vi "PI Id (FXP).vi"(5 "Process Value":fxp<+/-,32,4>, 7 "Setpoint":fxp<+/-,32,1>, 10 "Ki":fxp<+/-,32,4>, 11 "Kp":fxp<+/-,32,4>) -> (3 "Output":fxp<+/-,32,4> format="%.30g")   [LabVIEW 2025]
uses:
  <vilib>/rvi/FXPMathLib/FxpSub/XNode/nifxpmath_Sub.xnode
  <vilib>/rvi/FXPMathLib/sim/FxpSim.dll
  <vilib>/rvi/FXPMathLib/FxpMul/XNode/nifxpmath_Multiplier.xnode
  <vilib>/rvi/FXPMathLib/FxpAdd/XNode/nifxpmath_Add.xnode
panel:
  out "e*s":fxp<+/-,32,4> format="%.30g"
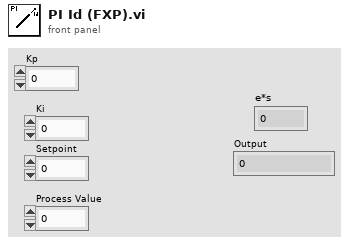
[diagram p1: front panel]
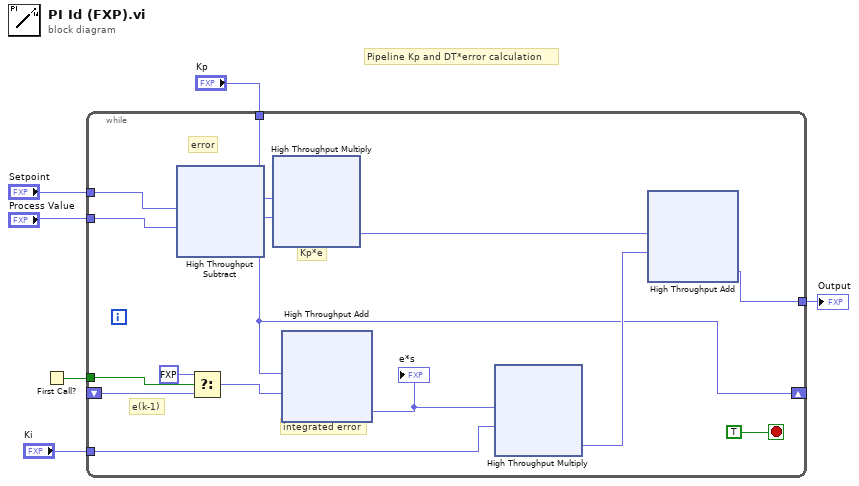
[diagram p0: block diagram]
diagram:
  # "Pipeline Kp and DT*error calculation"
  n1 = First Call?() -> (First Call?: T/F=w5:bool)
  n2 = while {
    shift-right: [w8] -> _
    shift-left: _ -> [w15]
    tunnel: w5 -> [w20]
    tunnel: "Setpoint" -> [w14]
    tunnel: "Process Value" -> [w13]
    tunnel: "Kp" -> [w12]
    tunnel: "Ki" -> [w10]
    tunnel: [w11] -> w6
    stop <- TRUE stop-if-true
    # "Kp*e"
    # "integrated error"
    # "e(k-1)"
    # "error"
    n3 = xnode "High Throughput Subtract"("x"=w14, "y"=w13) -> ("x-y"=w8:fxp<+/-,32,4>)
    n4 = Select(t=fxp<+/-,32,4> 0.0, s=w20, f=w15) -> (s? t:f=w9:fxp<+/-,32,4>)
    n5 = xnode "High Throughput Multiply"("x"=w12, "y"=w8) -> ("x*y"=w17:fxp<+/-,32,4>)
    n6 = xnode "High Throughput Add"("x"=w8, "y"=w9) -> ("x+y"=w7:fxp<+/-,32,4>)
    "e*s" <- w7
    n7 = xnode "High Throughput Multiply"("x"=w7, "y"=w10) -> ("x*y"=w16:fxp<+/-,32,4>)
    n8 = xnode "High Throughput Add"("x"=w17, "y"=w16) -> ("x+y"=w11:fxp<+/-,32,4>)
  }
  "Output" <- w6
